vi "controlAutoMeasure.vi"(7 "Set":bool, 8 "error in":errorcluster, 9 "enable":bool, 10 "axis in":u8, 11 "connection ID":refnum<k5>) -> (0 "error out":errorcluster, 1 "enable out":bool, 2 "axis out":i32, 3 "connection ID":refnum<k5>)   [LabVIEW 2016]
doc: "This function retrieves or sets the automatic C/R measurement on axis enable"
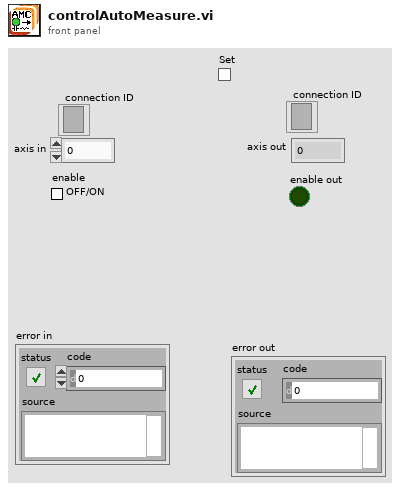
[diagram p1: front panel]
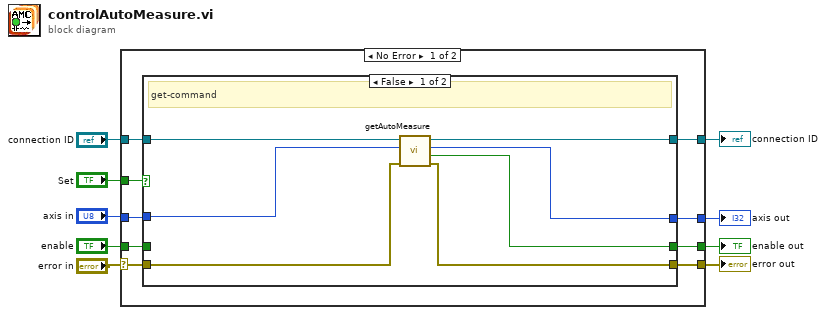
[diagram p0: block diagram]
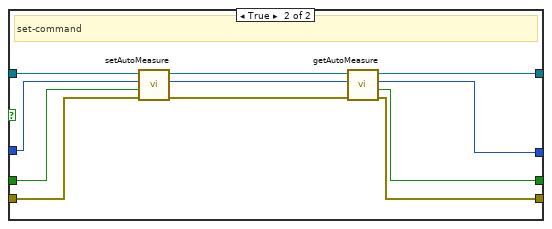
[diagram p2: hidden frame]
diagram:
  n1 = case shown="No Error" "error in" {
    selector: "error in" -> [w15 w40]
    tunnel: "axis in" -> [w18 w38]
    tunnel: [w13 w40] -> w8
    tunnel: "Set" -> [w16 _]
    tunnel: [w12 w39] -> w6
    tunnel: "connection ID" -> [w17 w39]
    tunnel: [w11 w38] -> w3
    tunnel: "enable" -> [w14 w37]
    tunnel: [w10 w37] -> w1
    frame No Error {
      n2 = case shown="False" w16 {
        tunnel: w17 -> [w23 w36]
        tunnel: w18 -> [w19 w35]
        tunnel: w15 -> [w25 w33]
        tunnel: w14 -> [_ w34]
        tunnel: [w24 w31] -> w13
        tunnel: [w22 w28] -> w12
        tunnel: [w21 w27] -> w11
        tunnel: [w20 w26] -> w10
        frame False {
          # "get-command"
          n3 = call "getAutoMeasure.vi"("error in"=w25, "axis"=w19, "connection ID"=w23) -> ("error out"=w24:errorcluster, "enable"=w20:bool, "axis_out"=w21:i32, "connection ID"=w22:refnum<k5>)  [unwired: 5 in]
        }
        frame True {
          # "set-command"
          n4 = call "setAutoMeasure.vi"("error in"=w33, "enable"=w34, "axis"=w35, "connection ID"=w36) -> ("error out"=w32:errorcluster, "axis_out"=w30:i32, "connection ID"=w29:refnum<k5>)  [unwired: 5 in]
          n5 = call "getAutoMeasure.vi"("error in"=w32, "axis"=w30, "connection ID"=w29) -> ("error out"=w31:errorcluster, "enable"=w26:bool, "axis_out"=w27:i32, "connection ID"=w28:refnum<k5>)  [unwired: 5 in]
        }
      }
    }
    frame Error {
    }
  }
  "error out" <- w8
  "axis out" <- w3
  "connection ID" <- w6
  "enable out" <- w1
